vi "testHeadersPresentParserSupport.vi"(8 "error in (no error)":errorcluster, 11 "reference in":refnum<class "EasyXML_XML_Subset_Built_Tests.lvclass">) -> (0 "error out":errorcluster, 3 "reference in":refnum<class "EasyXML_XML_Subset_Built_Tests.lvclass">)   [LabVIEW 2011, in "EasyXML_XML_Subset_Built_Tests.lvclass"]
uses:
  EasyXML_XML_Subset_Built_Tests.lvclass
  EasyXML_XML_Subset_Evaluations/EasyXML_XML_Subset_Evaluations.lvclass
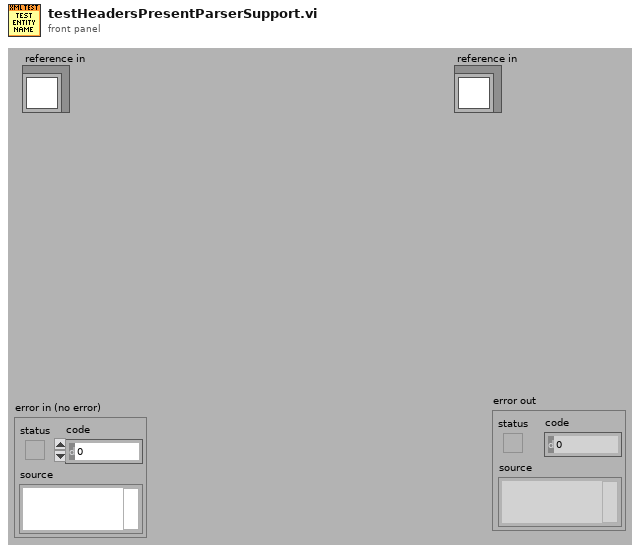
[diagram p1: front panel]
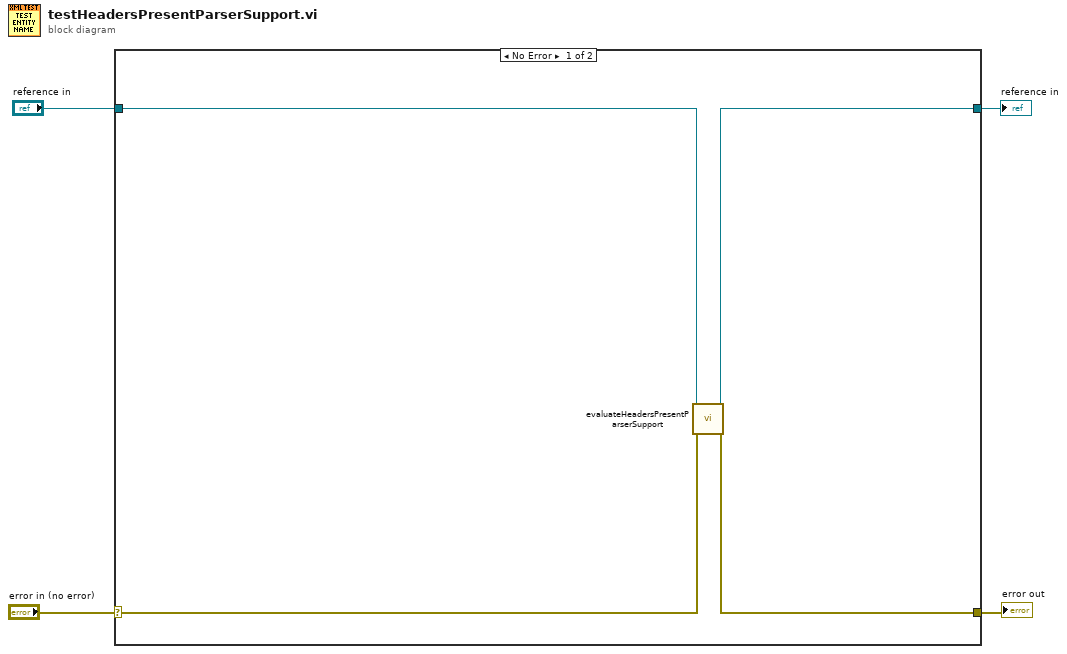
[diagram p0: block diagram]
diagram:
  n1 = case shown="No Error" "error in (no error)" {
    selector: "error in (no error)" -> [w6 w10]
    tunnel: [w5 w10] -> w3
    tunnel: [w7 w9] -> w1
    tunnel: "reference in" -> [w8 w9]
    frame No Error {
      n2 = call "evaluateHeadersPresentParserSupport.vi"("error in (no error)"=w6, "reference in"=w8) -> ("error out"=w5:errorcluster, "reference in"=w7:refnum<class "EasyXML_XML_Subset_Built_Tests.lvclass">)  [unwired: 8 in]
    }
    frame Error {
    }
  }
  "error out" <- w3
  "reference in" <- w1
